vi "fmt_formatTimestampStyles.vi"(7 "Columns":T1, 8 "error in":errorcluster) -> (0 "error out":errorcluster, 1 "styles map":string[](array[string]), 2 "cellXfs":string, 3 "numFmts":string)   [LabVIEW 2017, in "NI_ExcelFile.lvlib"]
uses:
  <vilib>/express/express shared/NI_ExcelFile/NI_ExcelFile.lvlib
  <vilib>/express/express shared/NI_ExcelFile/Ctrls/Columns.ctl
  <vilib>/express/express shared/NI_ExcelFile/Ctrls/ColumnInfo.ctl
  <vilib>/express/express shared/NI_ExcelFile/Ctrls/DataType.ctl
  <vilib>/express/express shared/NI_ExcelFile/SubVIs/fmt_getUTF-8Text.vi
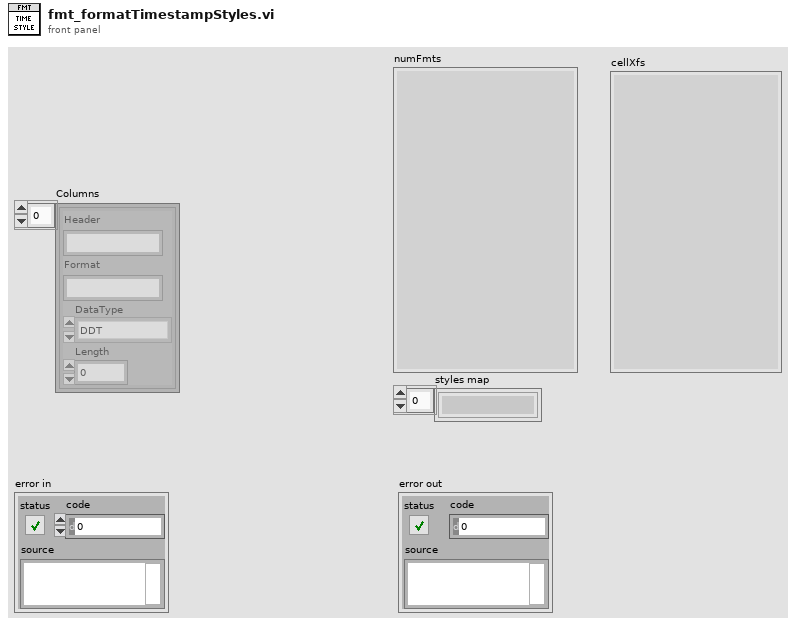
[diagram p1: front panel]
types:
  T1 = typedef "NI_ExcelFile.lvlib/Columns.ctl" = T2[]
  T2 = typedef "NI_ExcelFile.lvlib/ColumnInfo.ctl" = cluster{"Header":string, "Format":string, "DataType":T3, "Length":u64}
  T3 = typedef "NI_ExcelFile.lvlib/DataType.ctl" = enum16{"DDT", "WFM", "Array of STR", "Array of DBL", "Array of I8", "Array of I16", "Array of I32", "Array of I64", "Array of SGL", "Array of U8", "Array of U16", "Array of U32", "Array of U64", "Array of Time"}
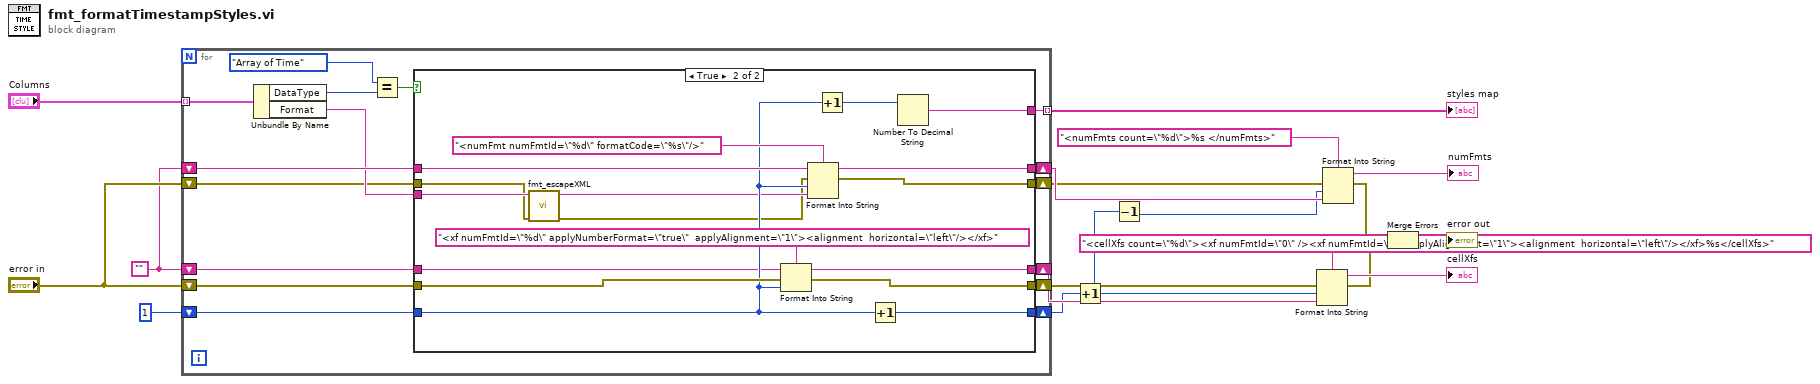
[diagram p0: block diagram]
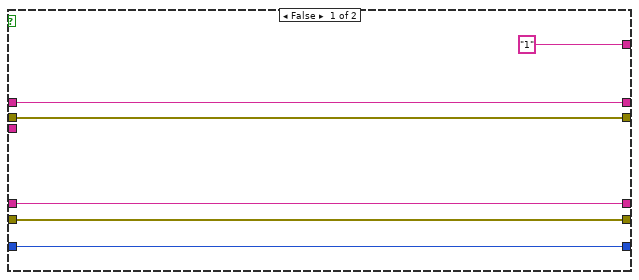
[diagram p2: hidden frame]
diagram:
  w12 = ""
  n1 = for {
    tunnel: "Columns" -> [w35] mode=indexing
    shift-right: [w31] -> w3
    shift-left: 1 -> [w33]
    tunnel: [w32] -> w14 mode=indexing
    shift-right: [w29] -> w10
    shift-left: w12 -> [w30]
    shift-right: [w27] -> w7
    shift-left: w12 -> [w28]
    shift-right: [w22] -> w9
    shift-left: "error in" -> [w23]
    shift-right: [w20] -> w6
    shift-left: "error in" -> [w21]
    n2 = Unbundle By Name(w35) -> ("DataType"=w26:T3, "Format"=w24:string)
    n3 = Equal?(x=DataType."Array of Time" ("y"), y=w26) -> (x = y?=w34:bool)
    n4 = case shown="True" w34 {
      tunnel: w33 -> [w40 w48]
      tunnel: ["1" w49] -> w32
      tunnel: [w40 w56] -> w31
      tunnel: w30 -> [w37 w47]
      tunnel: [w37 w57] -> w29
      tunnel: w28 -> [w38 w54]
      tunnel: [w38 w53] -> w27
      tunnel: w24 -> [_ w46]
      tunnel: w23 -> [w36 w52]
      tunnel: [w36 w51] -> w22
      tunnel: w21 -> [w39 w44]
      tunnel: [w39 w50] -> w20
      frame False {
      }
      frame True {
        n5 = call <vilib>:"fmt_escapeXML.vi"("error in"=w44, "plain text"=w46) -> ("error out"=w43:errorcluster, "xml text"=w45:string)  [unwired: 8 in]
        n6 = Format Into String(format string="<xf numFmtId=\"%d\" applyNumberFormat=\"true\"  applyAlignment=\"1\"><alignment  horizontal=\"left\"/></xf>", initial string=w47, error in=w52, w48) -> (resulting string=w57:string, error out=w51:errorcluster)
        n7 = Format Into String(format string="<numFmt numFmtId=\"%d\" formatCode=\"%s\"/>", initial string=w54, error in=w43, w48, w45) -> (resulting string=w53:string, error out=w50:errorcluster)
        n8 = Increment(x=w48) -> (x+1=w42:i32)
        n9 = Increment(x=w48) -> (x+1=w56:i32)
        n10 = Number To Decimal String(number=w42) -> (decimal integer string=w49:string)  [unwired: 1 in]
      }
    }
  }
  "styles map" <- w14
  n11 = Increment(x=w3) -> (x+1=w1:i32)
  n12 = Decrement(x=w3) -> (x-1=w2:i32)
  n13 = Format Into String(format string="<cellXfs count=\"%d\"><xf numFmtId=\"0\" /><xf numFmtId=\"0\" applyAlignment=\"1\"><alignment  horizontal=\"left\"/></xf>%s</cellXfs>", error in=w9, w1, w10) -> (resulting string=→"cellXfs":string, error out=w4:errorcluster)  [unwired: 1 in]
  n14 = Format Into String(format string="<numFmts count=\"%d\">%s </numFmts>", error in=w6, w2, w7) -> (resulting string=→"numFmts":string, error out=w5:errorcluster)  [unwired: 1 in]
  n15 = Merge Errors(w5, w4) -> (→"error out":errorcluster)
